vi "小三轮的 Motor.vi"(7 "Frequency":u16=50, 8 "错误输入（无错误）":errorcluster, 9 "Relay":bool=TRUE, 10 "PWM":dbl[](array[numeric])=[0.0, 0.0, 0.0, 0.0], 11 "Custom FPGA Reference Out":refnum<k20>) -> ()   [LabVIEW 2017]
uses:
  <vilib>/Utility/error.llb/Error Cluster From Error Code.vi
  <vilib>/rvi/errors/niLvFpgaAdjustHostInterfaceError.vi
  <vilib>/rvi/interface/nirviReadWriteControl/nirviReadWriteControl.xnode
  NiFpgaLv.dll
  <vilib>/rvi/interface/Simulation/niFpgaSimulationCallBeginRW.vi
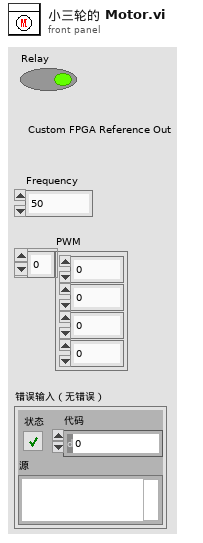
[diagram p1: front panel]
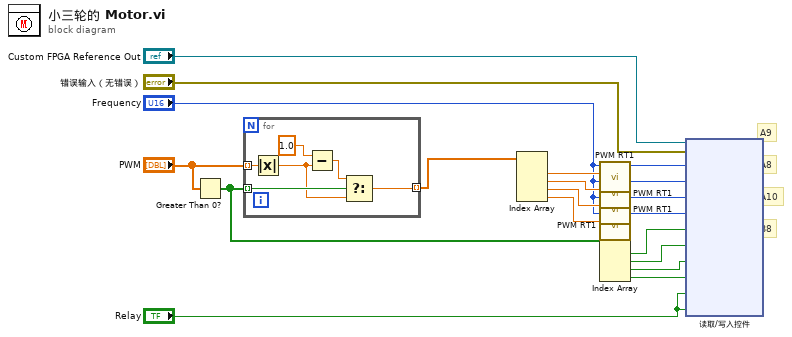
[diagram p0: block diagram]
diagram:
  # "A9"
  # "A10"
  # "A8"
  # "B8"
  n1 = Greater Than 0?(x="PWM") -> (x > 0?=w1:bool[])
  n2 = for {
    tunnel: "PWM" -> [w22] mode=indexing
    tunnel: w1 -> [w25] mode=indexing
    tunnel: [w21] -> w2 mode=indexing
    n3 = Absolute Value(x=w22) -> (abs(x)=w20:dbl)
    n4 = Subtract(x=1.0, y=w20) -> (x-y=w24:dbl)
    n5 = Select(t=w24, s=w25, f=w20) -> (s? t:f=w21:dbl)
  }
  n6 = Index Array(array=w2) -> (element #1=w9:dbl, element #2=w10:dbl, element #3=w11:dbl, element #4=w12:dbl)  [unwired: 4 in]
  n7 = call "PWM RT1.vi"("占空比"=w9, "频率"="Frequency") -> ("PWM FT"=w6:u32)  [unwired: 9 in]
  n8 = call "PWM RT1.vi"("占空比"=w10, "频率"="Frequency") -> ("PWM FT"=w5:u32)  [unwired: 9 in]
  n9 = call "PWM RT1.vi"("占空比"=w11, "频率"="Frequency") -> ("PWM FT"=w3:u32)  [unwired: 9 in]
  n10 = call "PWM RT1.vi"("占空比"=w12, "频率"="Frequency") -> ("PWM FT"=w4:u32)  [unwired: 9 in]
  n11 = Index Array(array=w1) -> (element #1=w14:bool, element #2=w15:bool, element #3=w16:bool, element #4=w17:bool)  [unwired: 4 in]
  n12 = xnode "读取/写入控件"("FPGA VI引用输入"="Custom FPGA Reference Out", "错误输入"="错误输入（无错误）", "PWM FT 1"=w6, "PWM FT 2"=w5, "PWM FT 3"=w3, "PWM FT 4"=w4, "DIR A9"=w14, "DIR A8"=w15, "DIR A10"=w16, "DIR B8"=w17, "Relay 4"="Relay", "Relay 13"="Relay") -> ()  [unwired: 2 out]
